vi "Dequeue.vi"(8 "Error In":errorcluster, 9 "timeout in ms (-1)":i32=-1, 11 "Queue in":refnum<queue>) -> (0 "Error Out":errorcluster, 1 "Data":variant, 2 "State":string, 3 "Queue out":refnum<queue>)   [LabVIEW 2019, in "Queues.lvlib"]
uses:
  Queues.lvlib
  Message Cluster.ctl
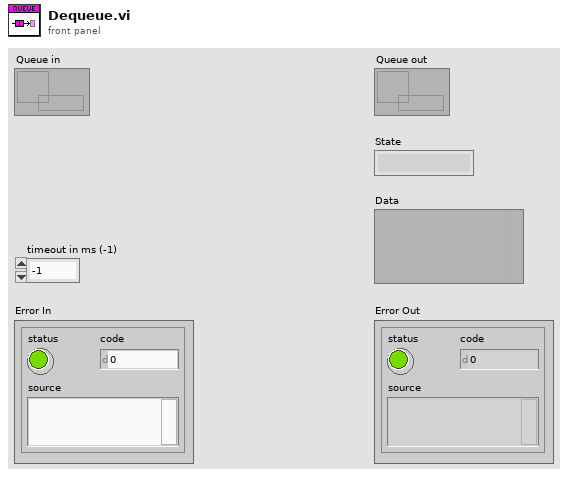
[diagram p1: front panel]
types:
  T1 = typedef "Queues.lvlib/Message Cluster.ctl" = cluster{"State":string, "Data":variant}
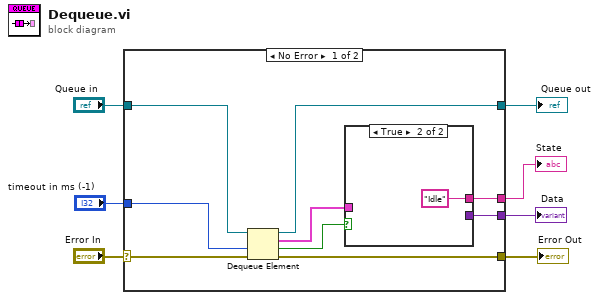
[diagram p0: block diagram]
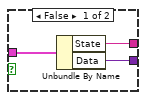
[diagram p2: hidden frame]
diagram:
  n1 = case shown="No Error" "Error In" {
    selector: "Error In" -> [w16 w22]
    tunnel: "Queue in" -> [w13 w21]
    tunnel: [w15 w22] -> w5
    tunnel: [w14 w21] -> w4
    tunnel: [w11 _] -> w3
    tunnel: [w10 _] -> w2
    tunnel: "timeout in ms (-1)" -> [w9 _]
    frame No Error {
      n2 = Dequeue Element(queue=w13, timeout in ms (-1)=w9, error in (no error)=w16) -> (queue out=w14:refnum<queue>, element=w12:T1, timed out?=w8:bool, error out=w15:errorcluster)
      n3 = case shown="True" w8 {
        tunnel: w12 -> [w19 _]
        tunnel: [w18 "Idle" ("State")] -> w11
        tunnel: [w17 _] -> w10
        frame False {
          n4 = Unbundle By Name(w19) -> ("State"=w18:string, "Data"=w17:variant)
        }
        frame True {
        }
      }
    }
    frame Error {
    }
  }
  "Error Out" <- w5
  "State" <- w3
  "Data" <- w2
  "Queue out" <- w4
